vi "CC FITS Write Housekeeping Values in FITS Header.vi"(8 "error in (no error)":errorcluster, 11 "gfits refnum":T1) -> (0 "error out":errorcluster, 3 "dup gfits refnum":T1)   [LabVIEW 2024]
uses:
  gfitsio/gfitsio-refnum.ctl
  Logging/CC enum Current Values Action.ctl
  gfitsio/gfitsio-write-key-double.vi
  gfitsio/gfitsio-write-key-string.vi
  hk-channel-class/hk-channel-class/HK Table/HK Table.lvclass
  gfitsio/gfitsio.lvlib
panel:
  in  "Detector #":u16
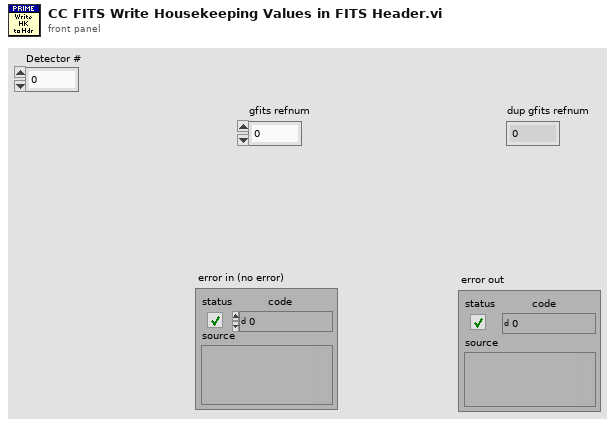
[diagram p1: front panel]
types:
  T1 = typedef "gfitsio.lvlib/gfitsio-refnum.ctl" = u64
  T2 = typedef "CC enum Current Values Action.ctl" = enum16{"Init", "Write Item", "Write Array", "Read Item", "Read Array", "Read All", "Add Channels", "New File", "Add Message", "Get Current Values", "Close"}
  T3 = typedef "FITS HK Header Table.ctl" = cluster{"Full Name":string, "FITS Name":string, "Units":string, "Comment":string}
  T4 = typedef "HK Item.lvclass/HK Channel Units and Setup.ctl" = cluster{"Unit Type":string, "Units":string, "Configuration":string, "Digits":i32, "Data Type":T5, "Exponential?":bool, "Source":string}
  T5 = typedef "HK Item.lvclass/HK Channel enum Data Type.ctl" = enum16{"Floating Point", "Integer", "Enum", "String", "Waveform", "File"}
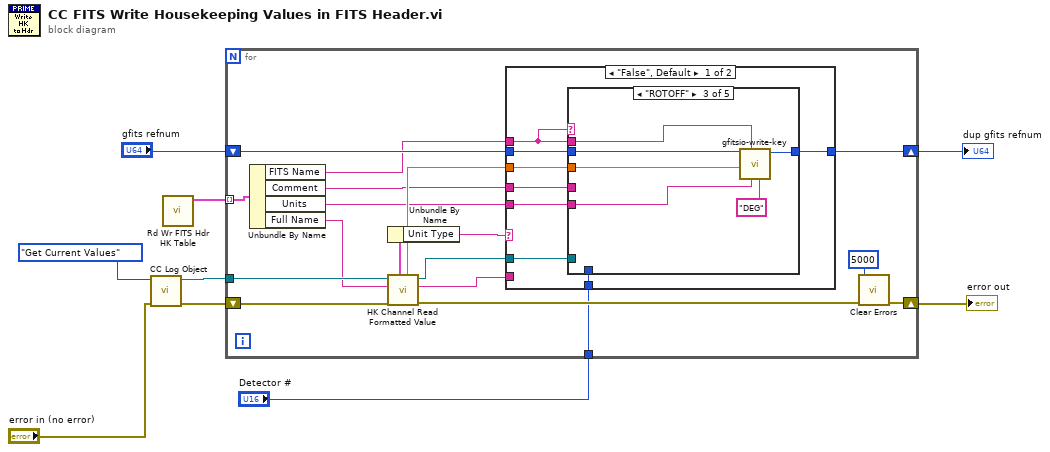
[diagram p0: block diagram]
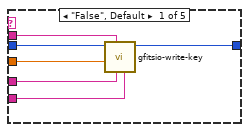
[diagram p2: hidden frame]
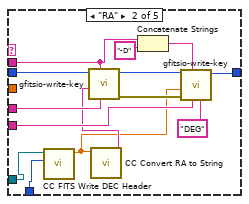
[diagram p3: hidden frame]
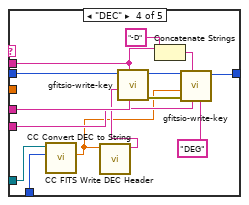
[diagram p4: hidden frame]
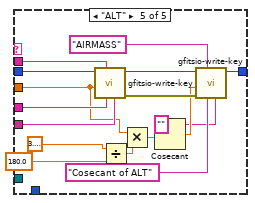
[diagram p5: hidden frame]
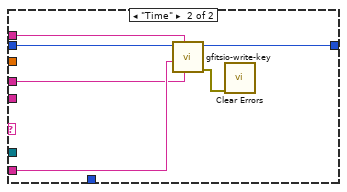
[diagram p6: hidden frame]
diagram:
  n1 = call "CC Log Object.vi"("error in (no error)"="error in (no error)", "Action"=CC_enum_Current_Values_Action."Get Current Values") -> ("error out"=w3:errorcluster, "HK Channel out"=w7:refnum<class "HK Table.lvclass">)  [unwired: 7 in, 1 out]
  n2 = call "Rd Wr FITS Hdr HK Table.vi"() -> ("FITS HK Hdr Table"=w8:T3[])  [unwired: 10 in, 1 out]
  n3 = for {
    tunnel: w8 -> [w27] mode=indexing
    tunnel: w7 -> [w26]
    shift-right: [w21] -> w5
    shift-left: "gfits refnum" -> [w24]
    shift-right: [w13] -> w2
    shift-left: w3 -> [w18]
    tunnel: "Detector #" -> [w10]
    n4 = Unbundle By Name(w27) -> ("FITS Name"=w23:string, "Comment"=w20:string, "Units"=w19:string, "Full Name"=w25:string)
    n5 = call-dynamic "HK Channel Read Formatted Value.vi"("error in (no error)"=w18, "Name"=w25, "HK Table.lvclass"=w26) -> ("error out"=w17:errorcluster, "Value Formatted"=w14:string, "HK Channel out"=w11:refnum<class "HK Table.lvclass">, "Value"=w22:dbl, "Channel Setup"=w16:T4)  [unwired: 1 in, 3 out]
    n6 = Unbundle By Name(w16) -> ("Unit Type"=w15:string)
    n7 = case shown="\"False\", Default" w15 {
      tunnel: w24 -> [w35 w97]
      tunnel: w23 -> [w30 w94]
      tunnel: w22 -> [w34 _]
      tunnel: [w33 w96] -> w21
      tunnel: w20 -> [w32 w93]
      tunnel: w19 -> [w31 _]
      tunnel: w14 -> [_ w95]
      tunnel: w11 -> [w29 _]
      tunnel: w10 -> [w28 _]
      frame "False", Default {
        n8 = case shown="\"ROTOFF\"" w30 {
          tunnel: w35 -> [w41 w55 w56 w75 w91]
          tunnel: w30 -> [w40 w51 w58 w71 w88]
          tunnel: w34 -> [w39 _ w57 _ w80]
          tunnel: [w38 w52 w61 w72 w84] -> w33
          tunnel: w32 -> [w37 w54 _ w74 w90]
          tunnel: w31 -> [w36 w47 w60 w67 w89]
          tunnel: w29 -> [_ w43 _ w64 _]
          tunnel: w28 -> [_ w44 _ w63 _]
          frame "False", Default {
            n9 = call-poly "gfitsio-write-key.vi"("units"=w36, "comment"=w37, "keyname"=w40, "value"=w39, "gfits refnum"=w41) -> ("dup gfits refnum"=w38:T1)  [unwired: 5 in, 1 out]
          }
          frame "RA" {
            n10 = call "CC FITS Write DEC Header.vi"("Detector #"=w44, "HK Channel"=w43) -> ("RA out"=w42:dbl)  [unwired: 7 in, 2 out]
            n11 = call "CC Convert RA to String.vi"("RA"=w42) -> ("RA String"=w46:string)  [unwired: 8 in, 2 out]
            n12 = call-poly "gfitsio-write-key.vi"("comment"=w54, "keyname"=w51, "value"=w46, "gfits refnum"=w55) -> ("error out"=w48:errorcluster, "dup gfits refnum"=w53:T1)  [unwired: 6 in]
            n13 = Concatenate Strings(w51, "-D" ("string")) -> (w49:string)
            n14 = call-poly "gfitsio-write-key.vi"("units"="DEG", "comment"=w47, "keyname"=w49, "error in (no error)"=w48, "value"=w42, "gfits refnum"=w53) -> ("dup gfits refnum"=w52:T1)  [unwired: 4 in, 1 out]
          }
          frame "ROTOFF" {
            n15 = call-poly "gfitsio-write-key.vi"("units"="DEG", "comment"=w60, "keyname"=w58, "value"=w57, "gfits refnum"=w56) -> ("dup gfits refnum"=w61:T1)  [unwired: 5 in, 1 out]
          }
          frame "DEC" {
            n16 = call "CC FITS Write DEC Header.vi"("Detector #"=w63, "HK Channel"=w64) -> ("DEC out"=w62:dbl)  [unwired: 7 in, 2 out]
            n17 = call "CC Convert DEC to String.vi"("DEC"=w62) -> ("DEC String"=w66:string)  [unwired: 8 in, 2 out]
            n18 = call-poly "gfitsio-write-key.vi"("comment"=w74, "keyname"=w71, "value"=w66, "gfits refnum"=w75) -> ("error out"=w68:errorcluster, "dup gfits refnum"=w73:T1)  [unwired: 6 in]
            n19 = Concatenate Strings(w71, "-D" ("string")) -> (w69:string)
            n20 = call-poly "gfitsio-write-key.vi"("units"="DEG", "comment"=w67, "keyname"=w69, "error in (no error)"=w68, "value"=w62, "gfits refnum"=w73) -> ("dup gfits refnum"=w72:T1)  [unwired: 4 in, 1 out]
          }
          frame "ALT" {
            n21 = call-poly "gfitsio-write-key.vi"("units"=w89, "comment"=w90, "keyname"=w88, "value"=w80, "gfits refnum"=w91) -> ("error out"=w86:errorcluster, "dup gfits refnum"=w87:T1)  [unwired: 5 in]
            n22 = Divide(x=3.141592653589793, y=180.0) -> (x/y=w81:dbl)
            n23 = Multiply(x=w80, y=w81) -> (x*y=w79:dbl)
            n24 = Cosecant(1:w79) -> (0:w78:dbl)
            n25 = call-poly "gfitsio-write-key.vi"("units"="", "comment"="Cosecant of ALT", "keyname"="AIRMASS", "error in (no error)"=w86, "value"=w78, "gfits refnum"=w87) -> ("dup gfits refnum"=w84:T1)  [unwired: 4 in, 1 out]
          }
        }
      }
      frame "Time" {
        n26 = call-poly "gfitsio-write-key.vi"("comment"=w93, "keyname"=w94, "value"=w95, "gfits refnum"=w97) -> ("error out"=w92:errorcluster, "dup gfits refnum"=w96:T1)  [unwired: 6 in]
        n27 = call <vilib>:"Clear Errors.vi"("error in (no error)"=w92) -> ()  [unwired: 5 in, 2 out]
      }
    }
    n28 = call <vilib>:"Clear Errors.vi"("error in (no error)"=w17, "specific error code to clear (0: all)"=5000) -> ("error out"=w13:errorcluster)  [unwired: 4 in, 1 out]
  }
  "error out" <- w2
  "dup gfits refnum" <- w5
